vi "Main.vi"(11 "Module Admin":refnum<class "Delacor_lib_QMH_Module Admin.lvclass">) -> ()   [LabVIEW 2020, in "UI.lvlib"]
doc: "This template is based off of the Queued Message Handler design pattern and the Queued Message Handler project template that ships with LabVIEW.\n\nThe main difference is that the queue is private to this module and communication between modules is performed via Broadcast and Request events.\n\nRequest events are wrapped in public API methods and are handled in the Event Handling Loop (EHL) of this VI. Any module can register for Broadcast events sent by this module. The EHL generates messages based on user interface actions.\n\nThe Message Handling Loop (MHL) processes messages generated by the EHL, or by other messages. The messages are string values, so new messages can be added easily to the Message Cases case structure in the MHL. Each message cluster can also provide an optional value for Message Data, which is a variant that can be converted to whatever message-specific data is required.\n_____\nBased on Delacor QMH Project Template 5.0.0.82."
uses:
  UI.lvlib
  <vilib>/Delacor/Delacor QMH/Libraries/Module Admin_class/Delacor_lib_QMH_Module Admin.lvclass
  Module Data--cluster.ctl
  <vilib>/Delacor/Delacor QMH/Libraries/Message Queue_class/Delacor_lib_QMH_Message Queue.lvclass/Delacor_lib_QMH_Message Queue.ctl
  Stop Argument--cluster.ctl
  <vilib>/Delacor/Delacor QMH/Libraries/Module Admin_class/Delacor_lib_QMH_Module Admin.lvclass/Delacor_lib_QMH_Module Admin.ctl
  <vilib>/Delacor/Delacor QMH/Libraries/Message Queue_class/Delacor_lib_QMH_Enqueue Message (Single).vi
  <vilib>/Delacor/Delacor QMH/Libraries/Module Admin_class/Delacor_lib_QMH_Get External Launch.vi
  <vilib>/Utility/error.llb/Error Cluster From Error Code.vi
  <vilib>/ErrorRing/Error Ring.xnode
  <vilib>/Delacor/Delacor QMH/Libraries/Message Queue_class/Delacor_lib_QMH_Message Queue.lvclass
  Productos/Productos.lvlib
  Mensajes/Mensajes.lvlib
  Monedas/Monedas.lvlib
  Config/Config.lvlib
panel:
  out "error out":errorcluster
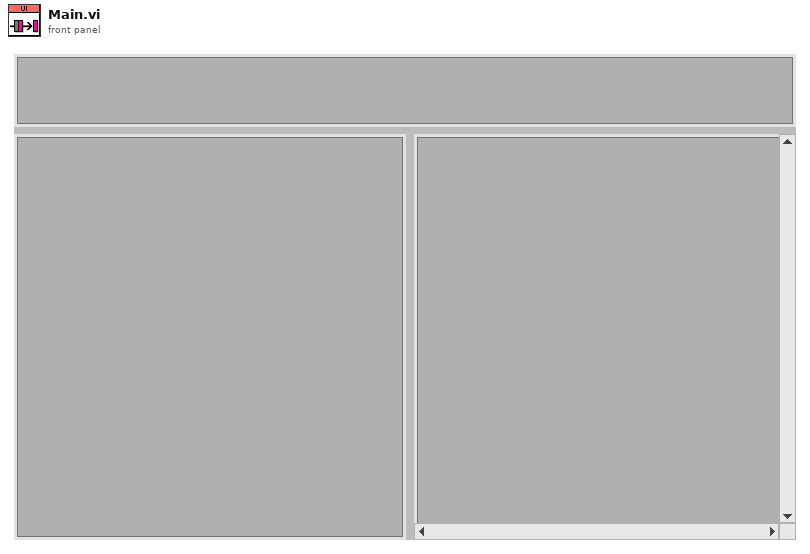
[diagram p1: front panel]
types:
  T1 = typedef "UI.lvlib/Request Events--cluster.ctl" = cluster{"Stop Module":refnum<user-event>, "Show Panel":refnum<user-event>, "Hide Panel":refnum<user-event>, "Get Module Execution Status":refnum<user-event>, "Show Diagram":refnum<user-event>}
  T2 = typedef "Productos.lvlib/Broadcast Events--cluster.ctl" = cluster{"Module Did Init":refnum<user-event>, "Status Updated":refnum<user-event>, "Error Reported":refnum<user-event>, "Module Did Stop":refnum<user-event>, "Update Module Execution Status":refnum<user-event>}
  T3 = typedef "Mensajes.lvlib/Broadcast Events--cluster.ctl" = cluster{"Module Did Init":refnum<user-event>, "Status Updated":refnum<user-event>, "Error Reported":refnum<user-event>, "Module Did Stop":refnum<user-event>, "Update Module Execution Status":refnum<user-event>}
  T4 = typedef "Config.lvlib/Broadcast Events--cluster.ctl" = cluster{"Module Did Init":refnum<user-event>, "Status Updated":refnum<user-event>, "Error Reported":refnum<user-event>, "Module Did Stop":refnum<user-event>, "Update Module Execution Status":refnum<user-event>}
  T5 = typedef "Monedas.lvlib/Broadcast Events--cluster.ctl" = cluster{"Module Did Init":refnum<user-event>, "Status Updated":refnum<user-event>, "Error Reported":refnum<user-event>, "Module Did Stop":refnum<user-event>, "Update Module Execution Status":refnum<user-event>}
  T6 = typedef "UI.lvlib/Module Data--cluster.ctl" = cluster{"Status":string}
  T7 = enum32{"invalid lock state", "Not Locked", "Locked (No Password)", "Password-protected"}
  T8 = typedef "UI.lvlib/Stop Argument--cluster.ctl" = cluster{"Origin":string, "Exit via Stop Module Req?":bool, "Wait for Module to stop?":bool}
  T9 = enum32{"Invalid", "Standard", "Closed", "Hidden", "Minimized", "Maximized"}
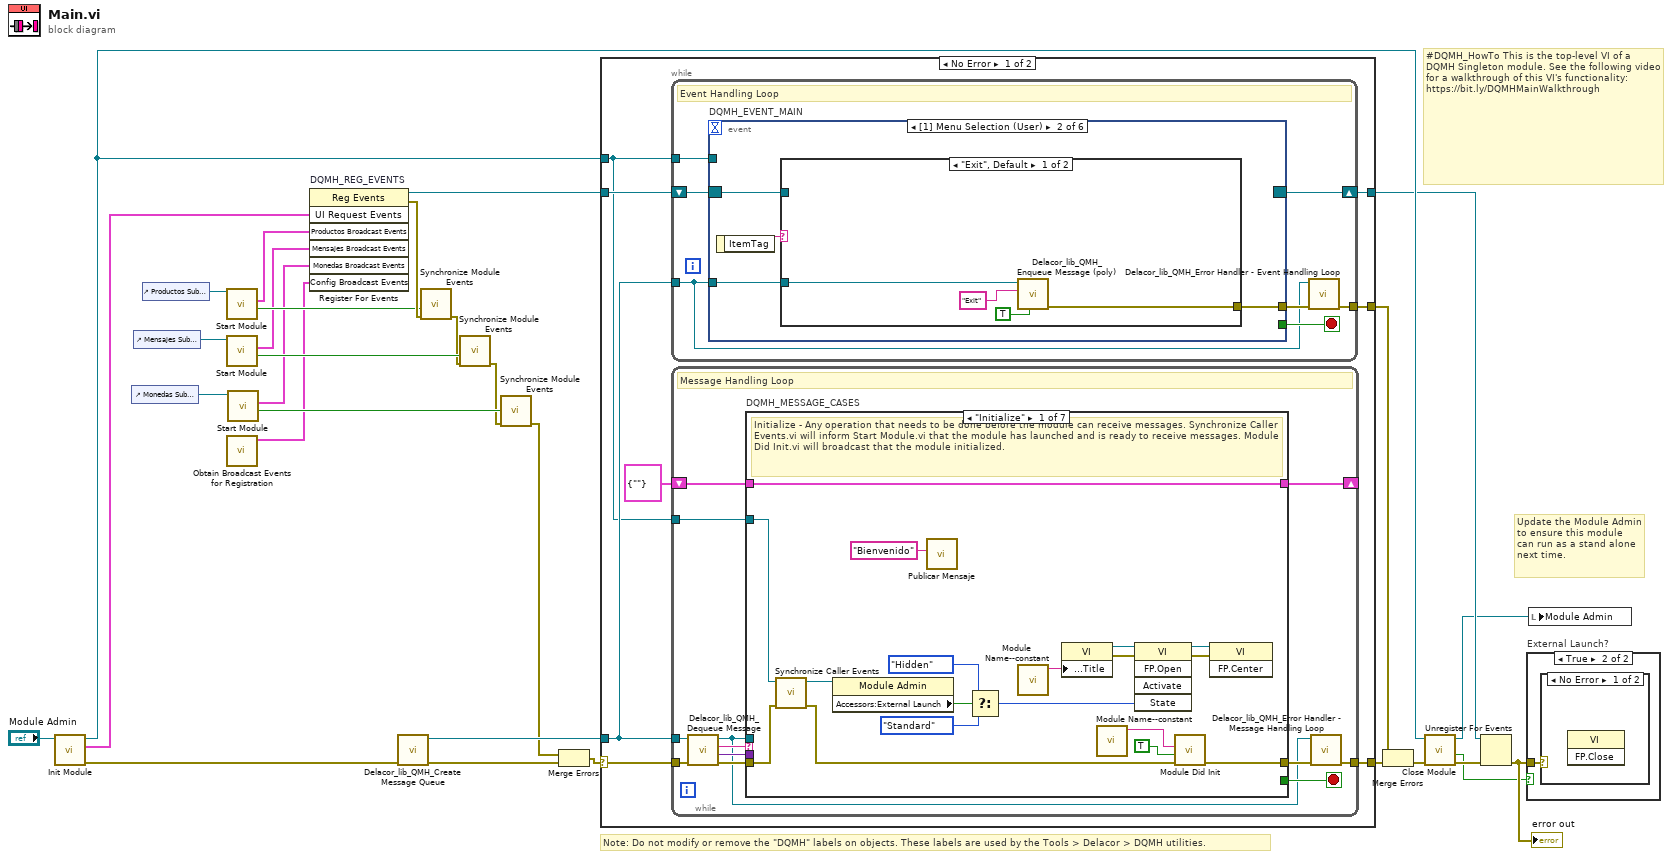
[diagram p0: block diagram]
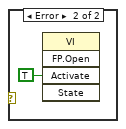
[diagram p3: hidden frame]
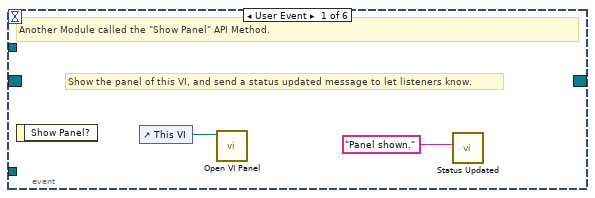
[diagram p4: hidden frame]
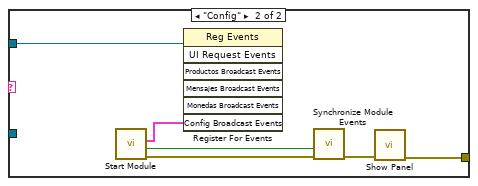
[diagram p5: hidden frame]
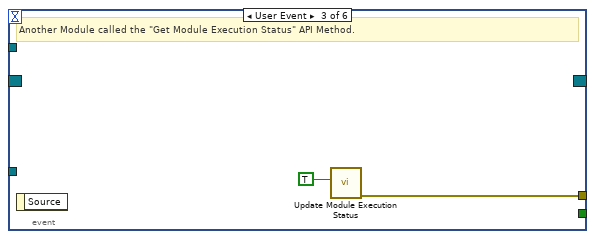
[diagram p6: hidden frame]
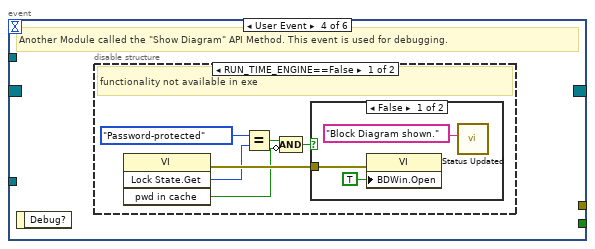
[diagram p7: hidden frame]
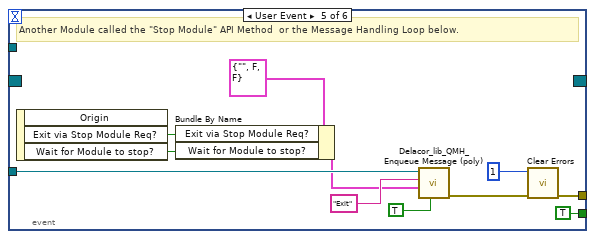
[diagram p10: hidden frame]
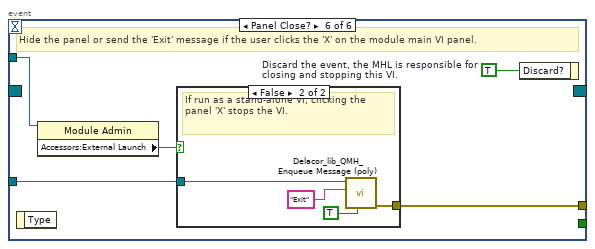
[diagram p11: hidden frame]
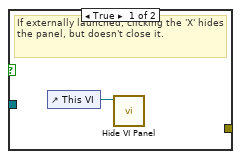
[diagram p12: hidden frame]
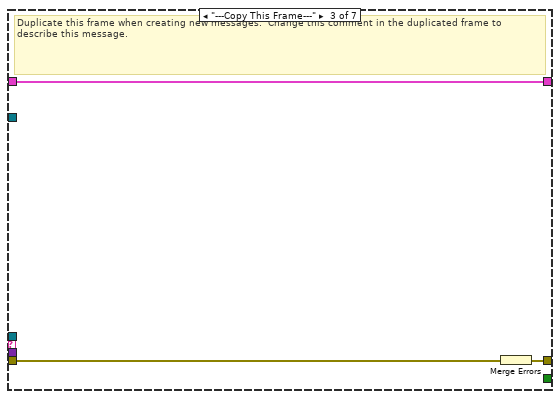
[diagram p14: hidden frame]
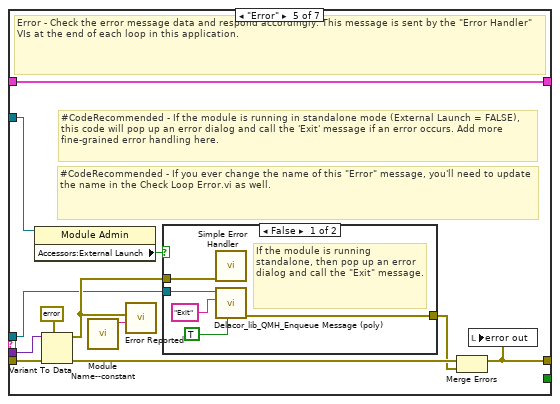
[diagram p16: hidden frame]
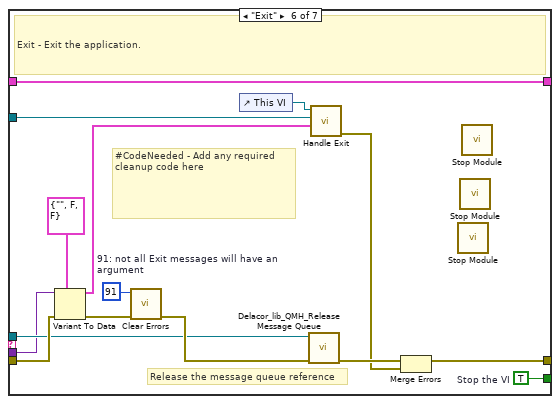
[diagram p18: hidden frame]
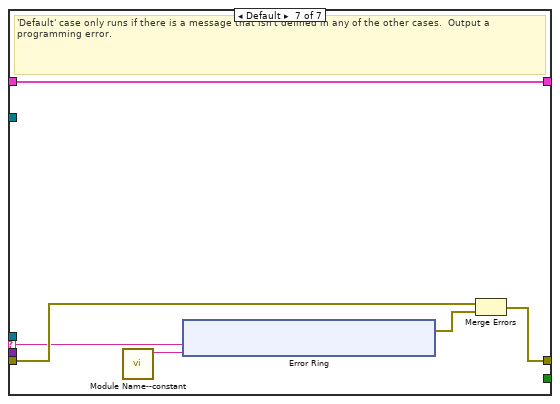
[diagram p19: hidden frame]
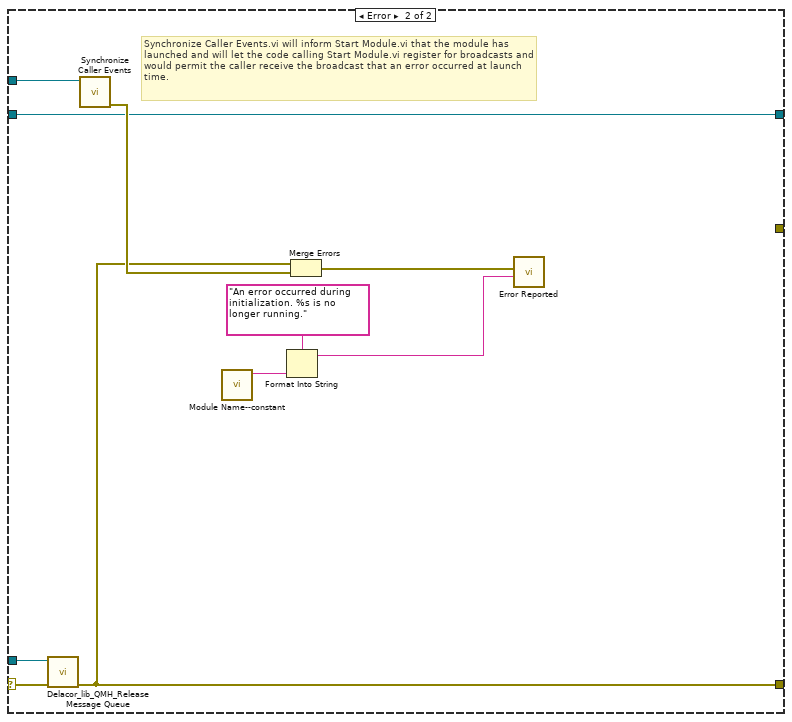
[diagram p20: hidden frame]
diagram:
  # "#DQMH_HowTo This is the top-level VI of a DQMH Singleton module. See the following video for a walkthrough of this VI's functionality: https://bit.ly/DQMHMainWalkthrough"
  # "Note: Do not modify or remove the \"DQMH\" labels on objects. These labels are used by the Tools > Delacor > DQMH utilities."
  # "Update the Module Admin to ensure this module can run as a stand alone next time."
  n1 = call "Init Module.vi"("Singleton Module Admin in"="Module Admin") -> ("error out"=w29:errorcluster, "UI Request Events"=w19:T1, "Singleton Module Admin out"=w22:refnum<class "Delacor_lib_QMH_Module Admin.lvclass">)  [unwired: 8 in]
  n2 = control-ref of="Monedas Sub Panel"() -> (w12:refnum<vi>)
  n3 = control-ref of="Mensajes Sub Panel"() -> (w13:refnum<vi>)
  n4 = control-ref of="Productos Sub Panel"() -> (w14:refnum<vi>)
  n5 = call "Start Module.vi"("Productos Sub Panel"=w14) -> ("Wait for Event Sync?"=w10:bool, "Productos Broadcast Events"=w7:T2)  [unwired: 7 in, 2 out]
  n6 = call "Start Module.vi"("Mensajes Sub Panel"=w13) -> ("Wait for Event Sync?"=w9:bool, "Mensajes Broadcast Events"=w6:T3)  [unwired: 7 in, 2 out]
  n7 = call "Obtain Broadcast Events for Registration.vi"() -> ("Config Broadcast Events"=w1:T4)  [unwired: 9 in, 2 out]
  n8 = call "Start Module.vi"("Monedas Sub Panel"=w12) -> ("Wait for Event Sync?"=w8:bool, "Monedas Broadcast Events"=w5:T5)  [unwired: 7 in, 2 out]
  n9 = register-events "DQMH_REG_EVENTS"(w19, w7, w6, w5, w1) -> (reference out=w20:refnum<event-registration>, error out=w11:errorcluster)  [unwired: 2 in]
  n10 = call <vilib>:"Delacor_lib_QMH_Create Message Queue.vi"("error in (no error)"=w29) -> ("error out"=w24:errorcluster, "Message Queue"=w18:refnum<class "Delacor_lib_QMH_Message Queue.lvclass">)  [unwired: 9 in]
  n11 = call "Synchronize Module Events.vi"("error in (no error)"=w11, "Wait for Event Sync?"=w10) -> ("error out"=w4:errorcluster)  [unwired: 9 in]
  n12 = call "Synchronize Module Events.vi"("error in (no error)"=w4, "Wait for Event Sync?"=w9) -> ("error out"=w3:errorcluster)  [unwired: 9 in]
  n13 = call "Synchronize Module Events.vi"("error in (no error)"=w3, "Wait for Event Sync?"=w8) -> ("error out"=w2:errorcluster)  [unwired: 9 in]
  n14 = Merge Errors(w2, w24) -> (w23:errorcluster)
  n15 = case shown="No Error" w23 {
    selector: w23 -> [w36 w179]
    tunnel: [w38 w178] -> w30
    tunnel: [w35 w184] -> w21
    tunnel: w20 -> [w33 w184]
    tunnel: w18 -> [w32 w177]
    tunnel: [w37 _] -> w27
    tunnel: w22 -> [w31 w180]
    frame No Error {
      n16 = while {
        tunnel: w32 -> [w39]
        shift-right: [w42] -> w35
        shift-left: w33 -> [w43]
        tunnel: [w44] -> w37
        tunnel: w31 -> [w40]
        stop <- w41 stop-if-true
        # "Event Handling Loop"
        n17 = event "DQMH_EVENT_MAIN" shown="[1] Menu Selection (User)" {
          selector: w43 -> [_ w50 _ _ _ _]
          dyn-events: [_ _ _ _ _ _] -> w42
          timeout: _ -> [_ _ _ _ _ _]
          tunnel: [_ _ _ _ TRUE ("Discard?") _] -> w41
          tunnel: w39 -> [_ w48 _ _ w79 w86]
          tunnel: [_ w49 w63 _ w82 w88] -> w45
          tunnel: w40 -> [_ _ _ _ _ w85]
          event User Event {
            # "Show the panel of this VI, and send a status updated message to let listeners know."
            # "Another Module called the \"Show Panel\" API Method."
            n18 = event-data() -> ()  [unwired: 1 in, 1 out]
            n19 = control-ref of="This VI"() -> (w47:refnum<vi>)
            n20 = call "Open VI Panel.vi"("VI"=w47) -> ()  [unwired: 10 in, 1 out]
            n21 = call "Status Updated.vi"("Status"="Panel shown." ("format string")) -> ()  [unwired: 10 in, 1 out]
          }
          event Menu Selection (User) {
            n22 = event-data() -> ("ItemTag"=w51:string)  [unwired: 1 in]
            n23 = case shown="\"Exit\", Default" w51 {
              tunnel: w50 -> [_ w61]
              tunnel: [w52 w60] -> w49
              tunnel: w48 -> [w53 _]
              frame "Exit", Default {
                n24 = call-poly <vilib>:"Delacor_lib_QMH_Enqueue Message (poly).vi"("Priority Message? (F)"=TRUE, "Message"="Exit", "Message Queue in"=w53) -> ("error out"=w52:errorcluster)  [unwired: 7 in, 1 out]
              }
              frame "Config" {
                n25 = call "Start Module.vi"() -> ("error out"=w58:errorcluster, "Wait for Event Sync?"=w57:bool, "Config Broadcast Events"=w56:T4)  [unwired: 8 in, 1 out]
                n26 = register-events(reference=w61, w56) -> ()  [unwired: 5 in, 2 out]
                n27 = call "Synchronize Module Events.vi"("error in (no error)"=w58, "Wait for Event Sync?"=w57) -> ("error out"=w59:errorcluster)  [unwired: 9 in]
                n28 = call "Show Panel.vi"("error in (no error)"=w59) -> ("error out"=w60:errorcluster)  [unwired: 10 in]
              }
            }
          }
          event User Event {
            # "Another Module called the \"Get Module Execution Status\" API Method."
            n29 = event-data() -> ()  [unwired: 1 in, 1 out]
            n30 = call "Update Module Execution Status.vi"("Running?"=TRUE) -> ("error out"=w63:errorcluster)  [unwired: 10 in]
          }
          event User Event {
            # "Another Module called the \"Show Diagram\" API Method. This event is used for debugging."
            n31 = event-data() -> ()  [unwired: 1 in, 1 out]
            n32 = disable-structure shown="RUN_TIME_ENGINE==False" {
              frame condition #0 (active) {
                # "functionality not available in exe"
                n33 = invoke class="VI" method="Lock State.Get"() -> (error out=w69:errorcluster, "Get Lock State"=w68:T7, "pwd in cache"=w65:bool)  [unwired: 4 in, 1 out]
                n34 = Equal?(x=T7."Password-protected", y=w68) -> (x = y?=w66:bool)
                n35 = Compound Arithmetic op=AND(w66, invert w65) -> (w64:bool)
                n36 = case shown="False" w64 {
                  tunnel: w69 -> [w72 _]
                  frame False {
                    n37 = property class="VI"(error in=w72, "BDWin.Open"=TRUE ("Block Diagram Window:Open")) -> ()  [unwired: 1 in, 2 out]
                    n38 = call "Status Updated.vi"("Status"="Block Diagram shown." ("format string")) -> ()  [unwired: 10 in, 1 out]
                  }
                  frame True {
                    # "Password-protected VI, and the password is not in the cache. Do not show the diagram."
                  }
                }
              }
              frame condition #1 {
              }
            }
          }
          event User Event {
            # "Another Module called the \"Stop Module\" API Method  or the Message Handling Loop below."
            n39 = event-data() -> ("Exit via Stop Module Req?"=w75:bool, "Wait for Module to stop?"=w74:bool)  [unwired: 1 in, 1 out]
            n40 = Bundle By Name(cluster=T8 {"Origin"="", "Exit via Stop Module Req?"=FALSE, "Wait for Module to stop?"=FALSE} ("Stop Argument"), "Exit via Stop Module Req?"=w75, "Wait for Module to stop?"=w74) -> (w73:T8)
            n41 = call-poly <vilib>:"Delacor_lib_QMH_Enqueue Message (poly).vi"("Priority Message? (F)"=TRUE, "Message Data"=w73, "Message"="Exit", "Message Queue in"=w79) -> ("error out"=w83:errorcluster)  [unwired: 6 in, 1 out]
            n42 = call <vilib>:"Clear Errors.vi"("error in (no error)"=w83, "specific error code to clear (0: all)"=1) -> ("error out"=w82:errorcluster)  [unwired: 4 in, 1 out]
          }
          event Panel Close? {
            w87 = TRUE  # Discard the event, the MHL is responsible for closing and stopping this VI.
            # "Hide the panel or send the 'Exit' message if the user clicks the 'X' on the module main VI panel."
            n43 = event-data() -> ()  [unwired: 1 in, 1 out]
            n44 = property class="Module Admin"(reference=w85) -> ("Accessors:External Launch"=w84:bool)  [unwired: 1 in, 2 out]
            n45 = case shown="False" w84 {
              tunnel: w86 -> [_ w92]
              tunnel: [_ w93] -> w88
              frame True {
                # "If externally launched, clicking the 'X' hides the panel, but doesn't close it."
                n46 = control-ref of="This VI"() -> (w89:refnum<vi>)
                n47 = call "Hide VI Panel.vi"("VI"=w89) -> ()  [unwired: 10 in, 1 out]
              }
              frame False {
                # "If run as a stand-alone VI, clicking the panel 'X' stops the VI."
                n48 = call-poly <vilib>:"Delacor_lib_QMH_Enqueue Message (poly).vi"("Priority Message? (F)"=TRUE, "Message"="Exit", "Message Queue in"=w92) -> ("error out"=w93:errorcluster)  [unwired: 7 in, 1 out]
              }
            }
            n49 = event-data("Discard?"=w87) -> ()  [unwired: 1 in, 1 out]
          }
        }
        n50 = call-dynamic "Delacor_lib_QMH_Error Handler - Event Handling Loop.vi"("error in (no error)"=w45, "Message Queue in"=w39) -> ("dup error in"=w44:errorcluster)  [unwired: 8 in, 1 out]
      }
      n51 = while {
        tunnel: w32 -> [w96]
        shift-right: [w100] -> _
        shift-left: T6 {"Status"=""} ("Data Cluster") -> [w101]
        tunnel: w36 -> [w104]
        tunnel: [w102] -> w38
        tunnel: w31 -> [w94]
        stop <- w99 stop-if-true
        # "Message Handling Loop"
        n52 = call-dynamic "Delacor_lib_QMH_Dequeue Message.vi"("error in (no error)"=w104, "Message Queue in"=w96) -> ("error out"=w103:errorcluster, "Message Data"=w97:variant, "Message"=w98:string, "Message Queue out"=w95:refnum<class "Delacor_lib_QMH_Message Queue.lvclass">)  [unwired: 6 in]
        n53 = case "DQMH_MESSAGE_CASES" shown="\"Initialize\"" w98 {
          selector: w98 -> [_ _ _ _ _ _ w164]
          tunnel: w95 -> [_ _ _ _ w134 w156 _]
          tunnel: w103 -> [w121 w125 w128 w130 w141 w162 w166]
          tunnel: [w119 w125 w127 w130 w137 w159 w167] -> w105
          tunnel: w101 -> [w110 w124 w126 w129 w136 w155 w165]
          tunnel: [w110 w124 w126 w129 w136 w155 w165] -> w100
          tunnel: [_ _ _ _ _ w154 _] -> w99
          tunnel: w97 -> [_ _ _ _ w135 w153 _]
          tunnel: w94 -> [w111 _ _ _ w133 w148 _]
          frame "Initialize" {
            # "Initialize - Any operation that needs to be done before the module can receive messages. Synchronize Caller Events.vi will inform Start Module.vi that the module has launched and is ready to receive messages. Module Did Init.vi will broadcast that the module initialized."
            n54 = call "Synchronize Caller Events.vi"("error in (no error)"=w121, "Singleton Module Admin in"=w111) -> ("error out"=w120:errorcluster, "Singleton Module Admin out"=w107:refnum<class "Delacor_lib_QMH_Module Admin.lvclass">)  [unwired: 8 in]
            n55 = property class="Module Admin"(reference=w107) -> ("Accessors:External Launch"=w115:bool)  [unwired: 1 in, 2 out]
            n56 = call "Publicar Mensaje.vi"("Mensaje"="Bienvenido") -> ()  [unwired: 10 in, 1 out]
            n57 = Select(t=T9."Hidden" ("State"), s=w115, f=T9."Standard" ("State")) -> (s? t:f=w112:T9)
            n58 = call "Module Name--constant.vi"() -> ("Module Name"=w118:string)  [unwired: 11 in]
            n59 = property class="VI"("Front Panel.Title"=w118) -> (reference out=w117:refnum<vi>, error out=w123:errorcluster)  [unwired: 2 in]
            n60 = call "Module Name--constant.vi"() -> ("Module Name"=w108:string)  [unwired: 11 in]
            n61 = invoke class="VI" method="FP.Open"(reference=w117, error in=w123, "State"=w112) -> (reference out=w116:refnum<vi>, error out=w122:errorcluster)  [unwired: 2 in, 3 out]
            n62 = call "Module Did Init.vi"("error in (no error)"=w120, "Initialized?"=TRUE, "Origin"=w108) -> ("error out"=w119:errorcluster)  [unwired: 8 in]
            n63 = invoke class="VI" method="FP.Center"(reference=w116, error in=w122) -> ()  [unwired: 1 in, 3 out]
          }
          frame "--- Module Specific ---" {
            # "Separator -- The following cases handle messages specific to this Module."
          }
          frame "---Copy This Frame---" {
            # "Duplicate this frame when creating new messages.  Change this comment in the duplicated frame to describe this message."
            n64 = Merge Errors(w128) -> (w127:errorcluster)
          }
          frame "--- Exit and Error Handling---" {
            # "Separator - The following cases handle errors and exit messages."
          }
          frame "Error" {
            # "#CodeRecommended - If you ever change the name of this \"Error\" message, you'll need to update the name in the Check Loop Error.vi as well."
            # "#CodeRecommended - If the module is running in standalone mode (External Launch = FALSE), this code will pop up an error dialog and call the 'Exit' message if an error occurs. Add more fine-grained error handling here."
            # "Error - Check the error message data and respond accordingly. This message is sent by the \"Error Handler\" VIs at the end of each loop in this application."
            n65 = property class="Module Admin"(reference=w133) -> ("Accessors:External Launch"=w132:bool)  [unwired: 1 in, 2 out]
            n66 = Variant To Data(error in=w141, type=errorcluster {"status"=FALSE, "code"=0, "source"=""} ("error constant"), Variant=w135) -> (data=w142:errorcluster, error out=w139:errorcluster)
            n67 = call "Module Name--constant.vi"() -> ("Module Name"=w131:string)  [unwired: 11 in]
            n68 = call "Error Reported.vi"("Additional Information"=w131, "Error"=w142) -> ()  [unwired: 9 in, 1 out]
            n69 = case shown="False" w132 {
              tunnel: [w147 _] -> w138
              tunnel: w134 -> [w145 _]
              tunnel: w142 -> [w146 _]
              frame False {
                # "If the module is running standalone, then pop up an error dialog and call the \"Exit\" message."
                n70 = call <vilib>:"Simple Error Handler.vi"("error in (no error)"=w146) -> ()  [unwired: 4 in, 5 out]
                n71 = call-poly <vilib>:"Delacor_lib_QMH_Enqueue Message (poly).vi"("Priority Message? (F)"=TRUE, "Message"="Exit", "Message Queue in"=w145) -> ("error out"=w147:errorcluster)  [unwired: 7 in, 1 out]
              }
              frame True {
                # "If the module was launched externally, calling the Error Reported broadcast VI is the only action performed by the \"Error\" message. The module's caller can then process the error appropriately."
              }
            }
            n72 = Merge Errors(w139, w138) -> (w137:errorcluster)
            n73 = local write "error out"(w137) -> ()
          }
          frame "Exit" {
            w152 = 91  # 91: not all Exit messages will have an argument
            w154 = TRUE  # Stop the VI
            # "Release the message queue reference"
            # "#CodeNeeded - Add any required cleanup code here"
            # "Exit - Exit the application."
            n74 = Variant To Data(error in=w162, type=T8 {"Origin"="", "Exit via Stop Module Req?"=FALSE, "Wait for Module to stop?"=FALSE} ("Stop Argument"), Variant=w153) -> (data=w150:T8, error out=w158:errorcluster)
            n75 = call <vilib>:"Clear Errors.vi"("error in (no error)"=w158, "specific error code to clear (0: all)"=w152) -> ("error out"=w161:errorcluster)  [unwired: 4 in, 1 out]
            n76 = control-ref of="This VI"() -> (w149:refnum<vi>)
            n77 = call-dynamic "Delacor_lib_QMH_Release Message Queue.vi"("error in (no error)"=w161, "Message Queue"=w156) -> ("error out"=w160:errorcluster)  [unwired: 9 in]
            n78 = call "Handle Exit.vi"("Stop Argument"=w150, "Admin in"=w148, "VI reference"=w149) -> ("error out"=w157:errorcluster)  [unwired: 7 in, 1 out]
            n79 = Merge Errors(w160, w157) -> (w159:errorcluster)
            n80 = call "Stop Module.vi"() -> ()  [unwired: 11 in, 1 out]
            n81 = call "Stop Module.vi"() -> ()  [unwired: 11 in, 1 out]
            n82 = call "Stop Module.vi"() -> ()  [unwired: 11 in, 1 out]
          }
          frame Default {
            # "'Default' case only runs if there is a message that isn't defined in any of the other cases.  Output a programming error."
            n83 = call "Module Name--constant.vi"() -> ("Module Name"=w163:string)  [unwired: 11 in]
            n84 = xnode "Error Ring"("parameter 0"=w164, "parameter 1"=w163) -> ("error out"=w168:errorcluster)
            n85 = Merge Errors(w166, w168) -> (w167:errorcluster)
          }
        }
        n86 = call-dynamic "Delacor_lib_QMH_Error Handler - Message Handling Loop.vi"("error in (no error)"=w105, "Message Queue in"=w95) -> ("dup error in"=w102:errorcluster)  [unwired: 8 in, 1 out]
      }
    }
    frame Error {
      # "Synchronize Caller Events.vi will inform Start Module.vi that the module has launched and will let the code calling Start Module.vi register for broadcasts and would permit the caller receive the broadcast that an error occurred at launch time."
      n87 = call-dynamic "Delacor_lib_QMH_Release Message Queue.vi"("error in (no error)"=w179, "Message Queue"=w177) -> ("error out"=w178:errorcluster)  [unwired: 9 in]
      n88 = call "Synchronize Caller Events.vi"("Singleton Module Admin in"=w180) -> ("error out"=w185:errorcluster)  [unwired: 9 in, 1 out]
      n89 = call "Module Name--constant.vi"() -> ("Module Name"=w183:string)  [unwired: 11 in]
      n90 = Format Into String(format string="An error occurred during initialization. %s is no longer running.", w183) -> (resulting string=w181:string)  [unwired: 2 in, 1 out]
      n91 = Merge Errors(w178, w185) -> (w186:errorcluster)
      n92 = call "Error Reported.vi"("Additional Information"=w181, "Error"=w186) -> ()  [unwired: 9 in, 1 out]
    }
  }
  n93 = Merge Errors(w27, w30) -> (w26:errorcluster)
  n94 = call "Close Module.vi"("error in (no error)"=w26, "Module Admin in"=w22) -> ("error out"=w28:errorcluster, "External Launch"=w15:bool, "Module Admin out"=w16:refnum<class "Delacor_lib_QMH_Module Admin.lvclass">)  [unwired: 7 in]
  n95 = Unregister For Events(event registration refnum=w21, error in=w28) -> (error out=w25:errorcluster)
  "error out" <- w25
  n96 = case "External Launch?" shown="True" w15 {
    tunnel: w25 -> [_ w187]
    frame False {
    }
    frame True {
      n97 = case shown="No Error" w187 {
        frame No Error {
          n98 = invoke class="VI" method="FP.Close"() -> ()  [unwired: 3 in, 3 out]
        }
        frame Error {
          n99 = invoke class="VI" method="FP.Open"("Activate"=TRUE ("Activate?")) -> ()  [unwired: 4 in, 5 out]
        }
      }
    }
  }
  n100 = local write "Module Admin"(w16) -> ()
